vi "Expand.vi"(8 "error in (no error)":errorcluster, 10 "ToExpand in":refnum<data-value>, 11 "MultiTree in":refnum<class "MultiTree.lvclass">) -> (0 "error out":errorcluster, 1 "ExpandedSearchNodes":refnum<data-value>[](array[refnum]), 2 "ToExpand out":refnum<data-value>, 3 "MultiTree out":refnum<class "MultiTree.lvclass">)   [LabVIEW 2014, in "MultiTree.lvlib" / "MultiTree.lvclass"]
uses:
  <userlib>/AdvancedDataStructures/ClassBased/MultiTree/MultiTree.lvclass
  <userlib>/AdvancedDataStructures/ClassBased/MultiTreeNode/MultiTreeNode.lvclass
  <userlib>/AdvancedDataStructures/ClassBased/MultiTreeNode/MultiTreeNode.lvclass/MultiTreeNode.ctl
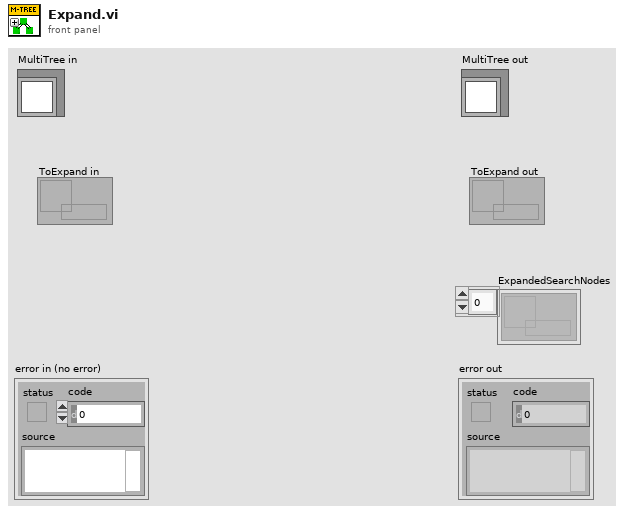
[diagram p1: front panel]
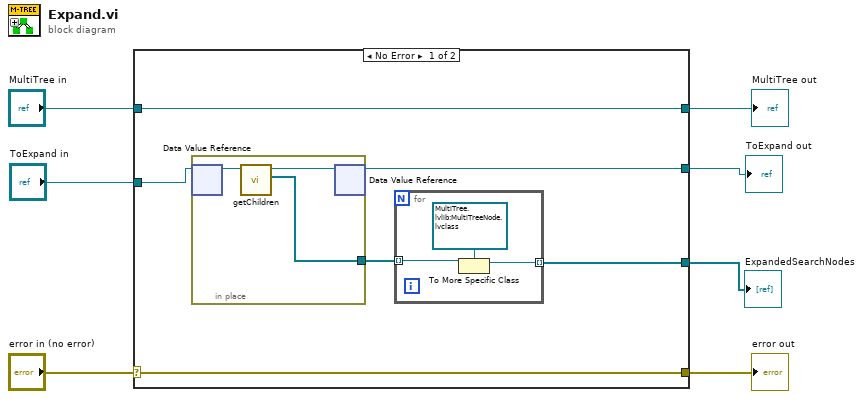
[diagram p0: block diagram]
diagram:
  n1 = case shown="No Error" "error in (no error)" {
    selector: "error in (no error)" -> [w12 w22]
    tunnel: [w12 w22] -> w6
    tunnel: [w13 w21] -> w4
    tunnel: "MultiTree in" -> [w13 w21]
    tunnel: "ToExpand in" -> [w10 w20]
    tunnel: [w9 w20] -> w2
    tunnel: [w8 _] -> w1
    frame No Error {
      n2 = in-place {
        in-place-border: [w17] -> w11
        n3 = in-place-dvr #1(w10) -> (w19:refnum<class "MultiTreeNode.lvclass">)  [unwired: 1 out]
        n4 = call <userlib>:"getChildren.vi"("MultiTreeNode in"=w19) -> ("Children"=w17:refnum<data-value>[], "MultiTreeNode out"=w18:refnum<class "MultiTreeNode.lvclass">)  [unwired: 8 in, 1 out]
        n5 = in-place-dvr #1(w18) -> (w9:refnum<data-value>)  [unwired: 1 out]
      }
      n6 = for {
        tunnel: w11 -> [w16] mode=indexing
        tunnel: [w14] -> w8 mode=indexing
        n7 = To More Specific Class(target class=refnum<data-value> refnum ("ToExpand in"), reference=w16) -> (specific class reference=w14:refnum<data-value>)  [unwired: 1 in, 1 out]
      }
    }
    frame Error {
    }
  }
  "error out" <- w6
  "MultiTree out" <- w4
  "ToExpand out" <- w2
  "ExpandedSearchNodes" <- w1
